vi "PATCH File.vi"(6 "timeout":i32=10000, 7 "output file":path, 8 "error in (no error)":errorcluster, 9 "file":path, 10 "url":string, 11 "HTTP Client Base in":refnum<class "LabVIEW HTTP Client.lvclass">) -> (0 "error out":errorcluster, 1 "body":string, 2 "headers":string, 3 "HTTP Client Base out":refnum<class "LabVIEW HTTP Client.lvclass">, 4 "status code":u32)   [LabVIEW 2020, in "HTTP Client Abstract.lvlib" / "LabVIEW HTTP Client.lvclass"]
uses:
  LabVIEW HTTP Client.lvclass
  Abstract HTTP Client/Abstract HTTP Client.lvclass
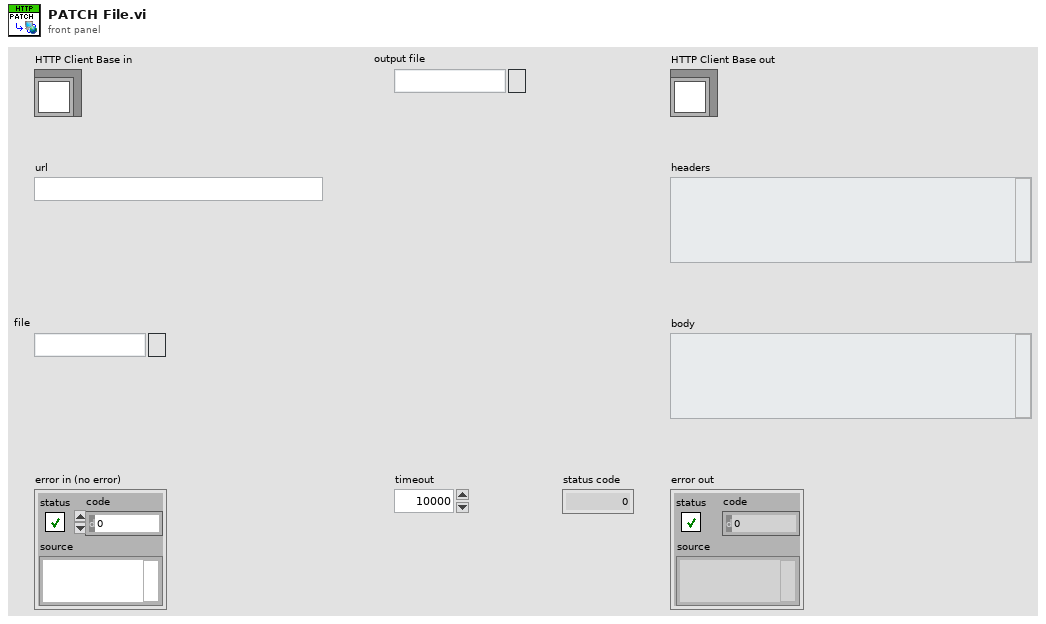
[diagram p1: front panel]
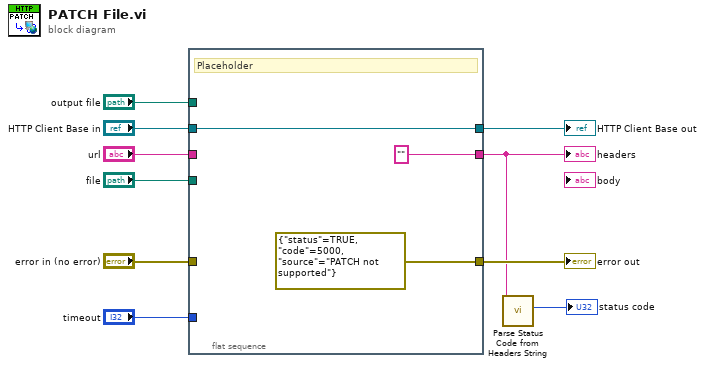
[diagram p0: block diagram]
diagram:
  n1 = flat-sequence {
    tunnel: [errorcluster {"status"=TRUE, "code"=5000, "source"="PATCH not supported"} ("error out")] -> w10
    tunnel: ["" ("headers")] -> w8
    tunnel: "timeout" -> [_]
    tunnel: "error in (no error)" -> [_]
    tunnel: "file" -> [_]
    tunnel: "url" -> [_]
    tunnel: "output file" -> [_]
    tunnel: [w11] -> w2
    tunnel: "HTTP Client Base in" -> [w11]
    frame #0 {
      # "Placeholder"
    }
  }
  n2 = call "Parse Status Code from Headers String.vi"("headers in"=w8) -> ("status code"=→"status code":u32)  [unwired: 10 in]
  "error out" <- w10
  "HTTP Client Base out" <- w2
  "headers" <- w8
